vi "pulse from memory 8spc_v3_host version.vi"(8 "run":bool=TRUE, 9 "referenses":T3={"clock x2"="IO Socket\\Data Clock 2x", "Memory In"="pulse on memory"}, 10 "start this pulse":bool, 11 "PDW":T1={"PW"=0, "frequency shift"=0.0, "amp"=0.9999923706054688, "mode type"=enum."CW", "mode depth"=0, "mode filter"=0, "phase shift"=0.0, "pulse shape filter"=0} {"frequency shift" format="%#_12f"}) -> (1 "free DDS":bool, 2 "output valid":bool=TRUE, 3 "IQ_out":T4[](array[typedef]))   [LabVIEW 2021]
uses:
  <instrlib>/_niInstr/DSP/v1/Shared/Public/IQ Data.ctl
  pdw.ctl
  CTL/mode_type.ctl
  <instrlib>/_niInstr/DSP/v1/FPGA/Public/Sub VIs/Data Conversion/U32 to IQ - 1 spc - S18.1.vi
  <instrlib>/FlexRIO/API/UsrFpgaDsp/v1/FPGA/HbInt/UsrFpgaDspHbIntIQ_8Cps_1xOC_BWper2_96dB.vi
  <instrlib>/FlexRIO/API/UsrFpgaDsp/v1/FPGA/HbInt/UsrFpgaDspHbIntIQ_4Cps_1xOC_BWper2_89dB.vi
  <instrlib>/FlexRIO/API/UsrFpgaDsp/v1/FPGA/HbInt/UsrFpgaDspHbIntIQ_2Cps_1xOC_BWper2_89dB.vi
  <instrlib>/FlexRIO/API/UsrFpgaDsp/v1/FPGA/HbInt/UsrFpgaDspHbIntIQ_1Spc_2xOC_BWper2_89dB.vi
  <instrlib>/FlexRIO/API/UsrFpgaDsp/v1/FPGA/HbInt/UsrFpgaDspHbIntIQ_2Spc_2xOC_BWper2_89dB.vi
  <instrlib>/FlexRIO/API/UsrFpgaDsp/v1/FPGA/HbInt/UsrFpgaDspHbIntIQ_4Spc_2xOC_BWper2_89dB.vi
  <instrlib>/FlexRIO/API/UsrFpgaDsp/v1/FPGA/HbInt/UsrFpgaDspHbIntIQ_8Spc_2xOC_BWper2_89dB.vi
  <instrlib>/_niInstr/DSP/v1/FPGA/Public/Sub VIs/Frequency Shift/Frequency Shift - 16 spc.vi
  <instrlib>/_niInstr/Basic Elements/v1/FPGA/Private/Count Up U32.vi
  <instrlib>/_niInstr/Basic Elements/v1/FPGA/Private/Count Up U16.vi
  <instrlib>/_niInstr/DSP/v1/Shared/niInstr DSP v1 Shared.lvlib
  <instrlib>/_niInstr/DSP/v1/FPGA/niInstr DSP v1 FPGA.lvlib
  <instrlib>/_niInstr/Basic Elements/v1/FPGA/niInstr Basic Elements v1 FPGA.lvlib
  <instrlib>/FlexRIO/API/UsrFpgaDsp/v1/FPGA/HbInt/UsrFpgaDsp HbInt v1 FPGA.lvlib
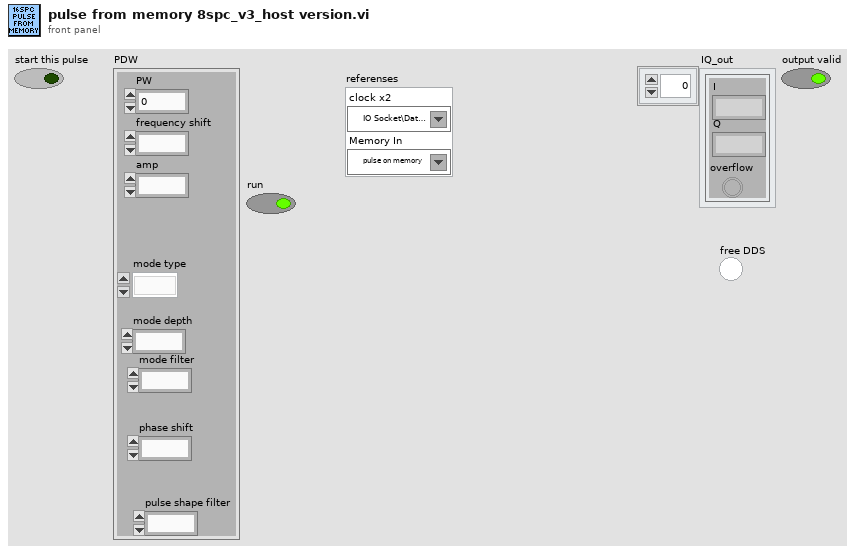
[diagram p1: front panel]
types:
  T1 = typedef "pdw.ctl" = cluster{"PW":u32, "frequency shift":fxp<+/-,48,0>, "amp":fxp<+/-,18,1>, "mode type":T2, "mode depth":u32, "mode filter":u8, "phase shift":fxp<+/-,16,1>, "pulse shape filter":u8}
  T2 = typedef "mode_type.ctl" = enum8{"CW", "from memory 1", "NC - cw", "LFM", "BPSK", "QPSK"}
  T3 = cluster{"clock x2":refnum<k21>, "Memory In":refnum<k21>}
  T4 = typedef "niInstr DSP v1 Shared.lvlib/IQ Data.ctl" = cluster{"I":fxp<+/-,18,1>, "Q":fxp<+/-,18,1>, "overflow":bool}
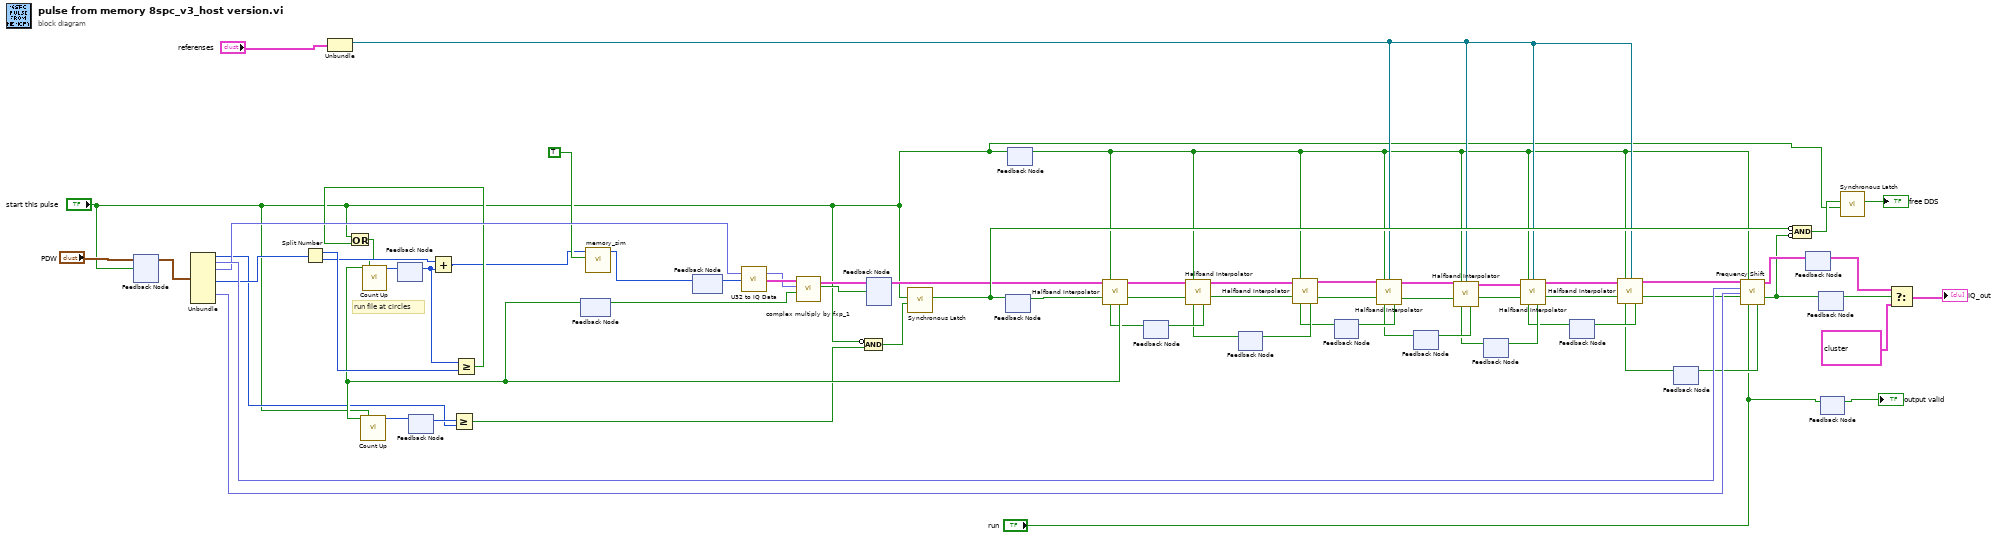
[diagram p0: block diagram]
diagram:
  # "run file at circles"
  n1 = feedback #1() -> (w63:T1)  [unwired: 1 in]
  n2 = feedback-in #1("PDW", "start this pulse") -> ()
  n3 = Unbundle(w63) -> ("PW"=w30:u32, "frequency shift"=w68:fxp<+/-,48,0>, "amp"=w57:fxp<+/-,18,1>, "mode depth"=w36:u32, "phase shift"=w67:fxp<+/-,16,1>)  [unwired: 3 out]
  n4 = Split Number(x=w36) -> (hi(x)=w62:u16, lo(x)=w56:u16)
  n5 = Unbundle("referenses") -> ("clock x2"=w26:refnum<k21>)  [unwired: 1 out]
  n6 = feedback #2() -> (w54:u16)  [unwired: 1 in]
  n7 = feedback #3() -> (w31:u32)  [unwired: 1 in]
  n8 = Add(x=w56, y=w54) -> (x+y=w6:u16)
  n9 = Greater Or Equal?(x=w31, y=w30) -> (x >= y?=w29:bool)
  n10 = Greater Or Equal?(x=w54, y=w62) -> (x >= y?=w33:bool)
  n11 = Or(x="start this pulse", y=w33) -> (x .or. y?=w34:bool)
  n12 = feedback #4() -> (w58:bool)  [unwired: 1 in]
  n13 = call "memory_sim.vi"("t-read;fwrite"=TRUE, "index"=w6) -> ("element out"=w8:u32)  [unwired: 8 in, 1 out]
  n14 = feedback #5() -> (w71:u32)  [unwired: 1 in]
  n15 = feedback-in #5(w8) -> ()
  n16 = call-poly <instrlib>:"U32 to IQ Data.vi"("U32 data"=w71) -> ("IQ data"=w60:T4)  [unwired: 14 in]
  n17 = call "complex multiply by fxp_1.vi"("input valid"=w58, "amp"=w57, "IQ data"=w60) -> ("data valid"=w61:bool, "output cluster"=w59:T4)  [unwired: 7 in]
  n18 = Compound Arithmetic op=AND(invert "start this pulse", w29) -> (w70:bool)
  n19 = feedback #6() -> (w38:T4)  [unwired: 1 in]
  n20 = feedback-in #6(w59, w61) -> ()
  n21 = call <instrlib>:"Synchronous Latch.vi"("clear"=w70, "set"="start this pulse") -> ("out"=w49:bool)  [unwired: 9 in]
  n22 = feedback #7() -> (w37:bool)  [unwired: 1 in]
  n23 = feedback-in #7(w49) -> ()
  n24 = feedback-in #8("start this pulse") -> ()
  n25 = feedback #8() -> (w25:bool)  [unwired: 1 in]
  n26 = feedback #9() -> (w21:bool)  [unwired: 1 in]
  n27 = call-poly "Halfband Interpolator.vi"("data in"=w38, "reset"=w25, "input valid"=w37, "ready for output (T)"=w21) -> ("data out"=w48:T4, "output valid"=w39:bool, "ready for input"=w32:bool)  [unwired: 9 in]
  n28 = call-poly <instrlib>:"Count Up.vi"("increment"=w32, "reset"="start this pulse") -> ("count out"=w35:u32)  [unwired: 13 in]
  n29 = call-poly <instrlib>:"Count Up.vi"("increment"=w32, "reset"=w34) -> ("count out"=w55:u16)  [unwired: 13 in]
  n30 = feedback-in #2(w55) -> ()
  n31 = feedback-in #3(w35) -> ()
  n32 = feedback-in #4(w32) -> ()
  n33 = feedback #10() -> (w19:bool)  [unwired: 1 in]
  n34 = call-poly "Halfband Interpolator.vi"("data in"=w48, "reset"=w25, "input valid"=w39, "ready for output (T)"=w19) -> ("data out"=w47:T4, "output valid"=w40:bool, "ready for input"=w22:bool)  [unwired: 9 in]
  n35 = feedback-in #9(w22) -> ()
  n36 = feedback #11() -> (w17:bool)  [unwired: 1 in]
  n37 = call-poly "Halfband Interpolator.vi"("data in"=w47, "reset"=w25, "input valid"=w40, "ready for output (T)"=w17) -> ("data out"=w46:T4, "output valid"=w41:bool, "ready for input"=w20:bool)  [unwired: 9 in]
  n38 = feedback-in #10(w20) -> ()
  n39 = feedback #12() -> (w15:bool)  [unwired: 1 in]
  n40 = call-poly "Halfband Interpolator.vi"("data in"=w46, "reset"=w25, "clk2x"=w26, "input valid"=w41, "ready for output (T)"=w15) -> ("data out"=w45:T4[], "output valid"=w42:bool, "ready for input"=w18:bool)  [unwired: 8 in]
  n41 = feedback-in #11(w18) -> ()
  n42 = feedback #13() -> (w13:bool)  [unwired: 1 in]
  n43 = call-poly "Halfband Interpolator.vi"("data in"=w45, "reset"=w25, "clk2x"=w26, "input valid"=w42, "ready for output (T)"=w13) -> ("data out"=w44:T4[], "output valid"=w43:bool, "ready for input"=w16:bool)  [unwired: 8 in]
  n44 = feedback-in #12(w16) -> ()
  n45 = feedback #14() -> (w11:bool)  [unwired: 1 in]
  n46 = call-poly "Halfband Interpolator.vi"("data in"=w44, "reset"=w25, "clk2x"=w26, "input valid"=w43, "ready for output (T)"=w11) -> ("data out"=w28:T4[], "output valid"=w27:bool, "ready for input"=w14:bool)  [unwired: 8 in]
  n47 = feedback-in #13(w14) -> ()
  n48 = feedback #15() -> (w9:bool)  [unwired: 1 in]
  n49 = call-poly "Halfband Interpolator.vi"("data in"=w28, "reset"=w25, "clk2x"=w26, "input valid"=w27, "ready for output (T)"=w9) -> ("data out"=w24:T4[], "output valid"=w23:bool, "ready for input"=w12:bool)  [unwired: 8 in]
  n50 = feedback-in #14(w12) -> ()
  n51 = call-poly <instrlib>:"Frequency Shift.vi"("data in"=w24, "reset"=w25, "frequency shift"=w68, "phase"=w67, "input valid"=w23, "ready for output (T)"="run") -> ("data out"=w53:T4[], "output valid"=w51:bool, "ready for input"=w10:bool)  [unwired: 6 in, 1 out]
  n52 = feedback-in #15(w10) -> ()
  n53 = Compound Arithmetic op=AND(invert w49, invert w51) -> (w3:bool)
  n54 = feedback #16() -> (w52:T4[])  [unwired: 1 in]
  n55 = feedback-in #16(w53) -> ()
  n56 = feedback #17() -> (w50:bool)  [unwired: 1 in]
  n57 = feedback-in #17(w51) -> ()
  n58 = feedback #18() -> (→"output valid":bool)  [unwired: 1 in]
  n59 = feedback-in #18("run") -> ()
  n60 = call <instrlib>:"Synchronous Latch.vi"("clear"="start this pulse", "set"=w3) -> ("out"=→"free DDS":bool)  [unwired: 9 in]
  n61 = Select(t=w52, s=w50, f=T4[] [{"I"=0.0, "Q"=0.0, "overflow"=FALSE}, {"I"=0.0, "Q"=0.0, "overflow"=FALSE}, {"I"=0.0, "Q"=0.0, "overflow"=FALSE}, {"I"=0.0, "Q"=0.0, "overflow"=FALSE}, {"I"=0.0, "Q"=0.0, "overflow"=FALSE}, {"I"=0.0, "Q"=0.0, "overflow"=FALSE}, {"I"=0.0, "Q"=0.0, "overflow"=FALSE}, {"I"=0.0, "Q"=0.0, "overflow"=FALSE}, {"I"=0.0, "Q"=0.0, "overflow"=FALSE}, {"I"=0.0, "Q"=0.0, "overflow"=FALSE}, {"I"=0.0, "Q"=0.0, "overflow"=FALSE}, {"I"=0.0, "Q"=0.0, "overflow"=FALSE}, {"I"=0.0, "Q"=0.0, "overflow"=FALSE}, {"I"=0.0, "Q"=0.0, "overflow"=FALSE}, {"I"=0.0, "Q"=0.0, "overflow"=FALSE}, {"I"=0.0, "Q"=0.0, "overflow"=FALSE}] ("data out")) -> (s? t:f=→"IQ_out":T4[])
